vi "DestroyPrivateEvents.vi"(8 "error in (no error)":errorcluster, 11 "Inst.TC":refnum<class "Inst.TC.lvclass">) -> (0 "error out":errorcluster, 3 "Inst.TC out":refnum<class "Inst.TC.lvclass">)   [LabVIEW 2019, in "Inst.TC.lvclass"]
doc: "JKI State Machine Objects (SMO) 1.0.0.5\nJKI - JKI\nCopyright (c) 2016, JKI"
uses:
  Inst.TC.lvclass
  Inst.TC.lvclass/Inst.TC.ctl
  <userlib>/LevyLab/Instrument Framework/Instrument Types/Cryostat/Instrument.Cryostat.lvclass
panel:
  # "For instructions on how to use the JKI State Machine Objects, examples and video tutorials, visit:\nhttp://jki.net/state-machine-objects/\n\nJKI State Machine Objects™\nhttp://jki.net/state-machine-objects/\nCopyright (C) 2005-2015, JKI <info@jki.net>\nALL RIGHTS RESERVED"
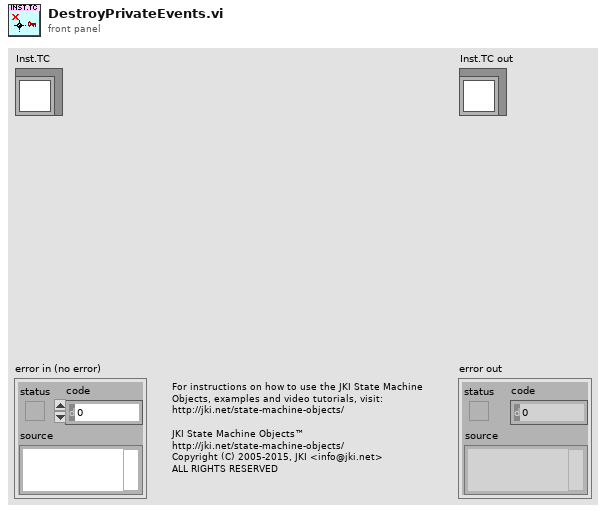
[diagram p1: front panel]
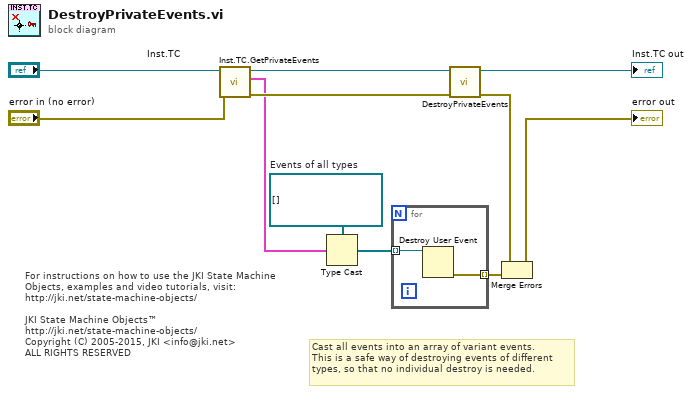
[diagram p0: block diagram]
diagram:
  w8 = refnum<user-event>[] []  # Events of all types
  # "For instructions on how to use the JKI State Machine Objects, examples and video tutorials, visit:\nhttp://jki.net/state-machine-objects/\n\nJKI State Machine Objects™\nhttp://jki.net/state-machine-objects/\nCopyright (C) 2005-2015, JKI <info@jki.net>\nALL RIGHTS RESERVED"
  # "Cast all events into an array of variant events.\nThis is a safe way of destroying events of different\ntypes, so that no individual destroy is needed."
  n1 = call "Inst.TC.GetPrivateEvents.vi"("error in (no error)"="error in (no error)", "Inst.TC in"="Inst.TC") -> ("error out"=w2:errorcluster, "Inst.TC Private Events"=w1:cluster{"MessageToProcess":refnum<user-event>}, "Inst.TC out"=w4:refnum<class "Inst.TC.lvclass">)  [unwired: 7 in]
  n2 = Type Cast(type=w8, x=w1) -> (*(type *) &x=w9:refnum<user-event>[])
  n3 = for {
    tunnel: w9 -> [w13] mode=indexing
    tunnel: [w12] -> w7 mode=indexing
    n4 = Destroy User Event(user event=w13) -> (error out=w12:errorcluster)  [unwired: 1 in]
  }
  n5 = call-parent "DestroyPrivateEvents.vi"("error in (no error)"=w2, "Instrument"=w4) -> ("error out"=w5:errorcluster, "Instrument out"=→"Inst.TC out":refnum<class "Inst.TC.lvclass">)  [unwired: 8 in]
  n6 = Merge Errors(w5, w7) -> (→"error out":errorcluster)
